vi "Wait for Response Message.vi"(8 "error in (no error)":errorcluster, 9 "timeout in ms":i32, 11 "Process in":refnum<class "Process.lvclass">) -> (0 "error out":errorcluster, 1 "Message Data":variant, 2 "Message":string, 3 "Process out":refnum<class "Process.lvclass">, 4 "timed out?":bool)   [LabVIEW 2020, in "Process.lvclass"]
uses:
  Process.lvclass
  Process.lvclass/Process.ctl
  <vilib>/Utility/error.llb/Error Cluster From Error Code.vi
  <vilib>/ErrorRing/Error Ring.xnode
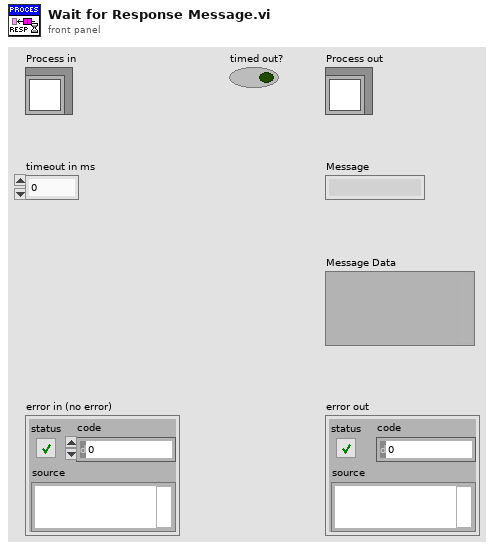
[diagram p1: front panel]
types:
  T1 = typedef "Process.lvclass/Lifecycle State.ctl" = enum16{"Uninitialized", "Initialized", "Started", "Running", "Stopped", "Finished"}
  T2 = typedef "Process.lvclass/Request Message Cluster.ctl" = cluster{"Message":string, "Message Data":variant}
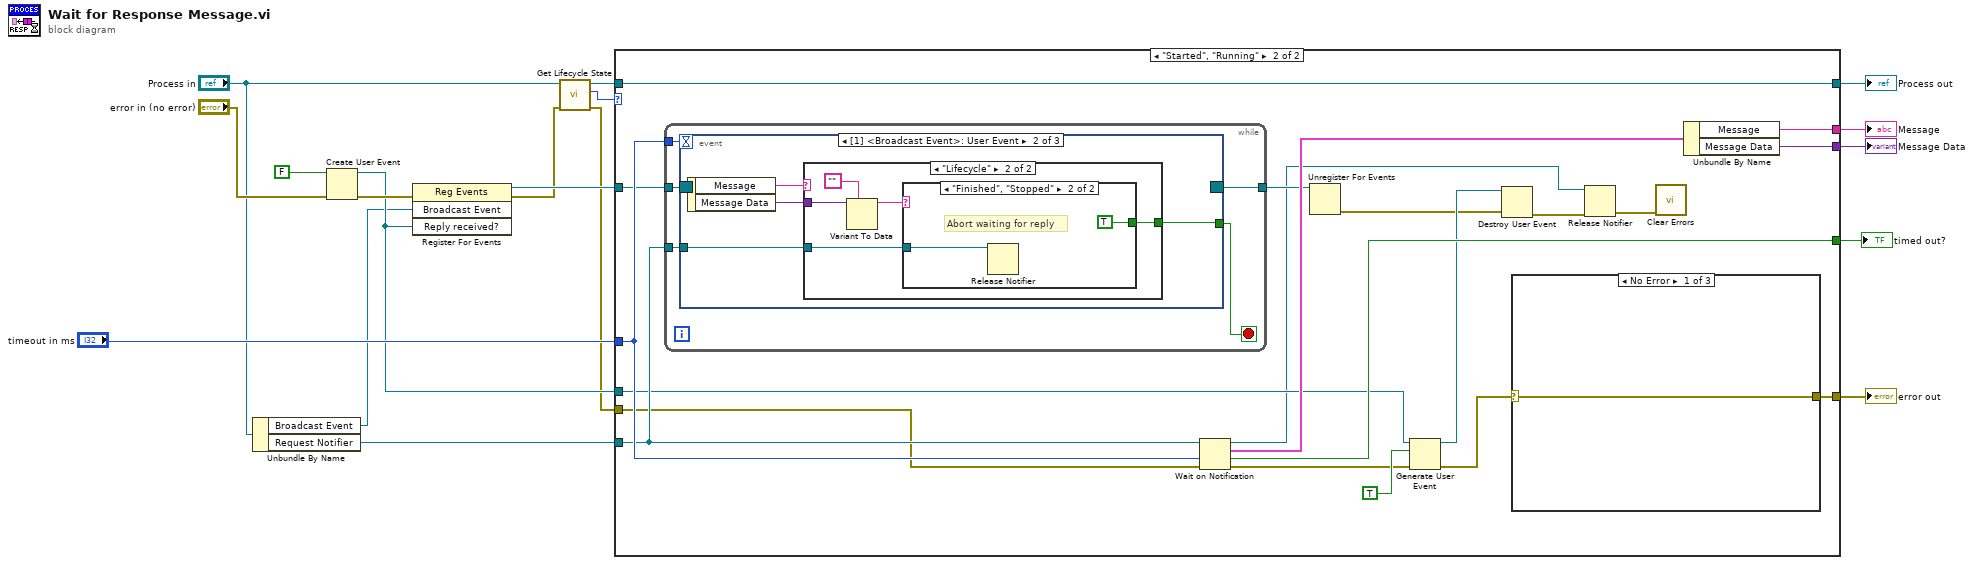
[diagram p0: block diagram]
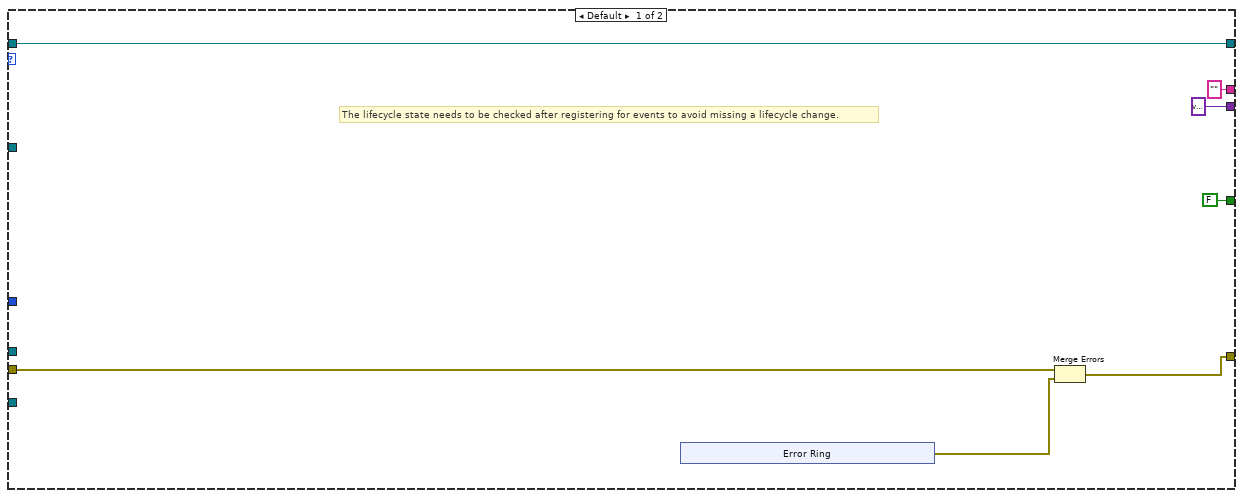
[diagram p2: hidden frame]
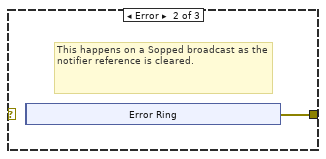
[diagram p3: hidden frame]
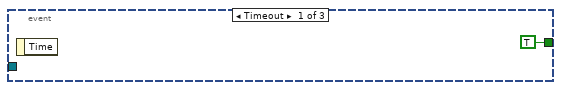
[diagram p5: hidden frame]
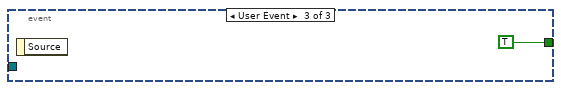
[diagram p8: hidden frame]
diagram:
  n1 = Unbundle By Name("Process in") -> ("Broadcast Event"=w6:refnum<user-event>, "Request Notifier"=w9:refnum<notifier>)
  n2 = Create User Event(user event datatype=FALSE ("Reply received?"), error in="error in (no error)") -> (user event=w7:refnum<user-event>, error out=w17:errorcluster)
  n3 = register-events(error in=w17, w6, w7) -> (reference out=w14:refnum<event-registration>, error out=w5:errorcluster)  [unwired: 1 in]
  n4 = call "Get Lifecycle State.vi"("error in (no error)"=w5, "Process In"="Process in") -> ("error out"=w4:errorcluster, "Lifecycle State"=w1:T1, "Process Out"=w2:refnum<class "Process.lvclass">)  [unwired: 6 in, 1 out]
  n5 = case shown="\"Started\", \"Running\"" w1 {
    tunnel: "timeout in ms" -> [_ w49]
    tunnel: w14 -> [_ w48]
    tunnel: [variant ("Message Data") w47] -> w13
    tunnel: ["" ("Message") w46] -> w12
    tunnel: [FALSE ("timed out?") w44] -> w11
    tunnel: w9 -> [_ w43]
    tunnel: [w23 w41] -> w8
    tunnel: w7 -> [_ w39]
    tunnel: w4 -> [w24 w31]
    tunnel: [w25 w30] -> w3
    tunnel: w2 -> [w25 w30]
    frame Default {
      # "The lifecycle state needs to be checked after registering for events to avoid missing a lifecycle change."
      n6 = xnode "Error Ring"() -> ("error out"=w22:errorcluster)
      n7 = Merge Errors(w24, w22) -> (w23:errorcluster)
    }
    frame "Started", "Running" {
      n8 = while {
        tunnel: w48 -> [w65]
        tunnel: w49 -> [w64]
        tunnel: w43 -> [w62]
        tunnel: [w61] -> w42
        stop <- w63 stop-if-true
        n9 = event shown="[1] <Broadcast Event>: User Event" {
          selector: w65 -> [_ _ _]
          dyn-events: [_ _ _] -> w61
          timeout: w64 -> [_ _ _]
          tunnel: [TRUE w67 TRUE] -> w63
          tunnel: w62 -> [_ w68 _]
          event Timeout {
            n10 = event-data() -> ()  [unwired: 1 in, 1 out]
          }
          event User Event {
            n11 = event-data() -> ("Message"=w70:string, "Message Data"=w69:variant)  [unwired: 1 in]
            n12 = case shown="\"Lifecycle\"" w70 {
              tunnel: w69 -> [_ w75]
              tunnel: w68 -> [_ w72]
              tunnel: [_ w71] -> w67
              frame Default {
              }
              frame "Lifecycle" {
                n13 = Variant To Data(type="", Variant=w75) -> (data=w73:string)  [unwired: 1 in, 1 out]
                n14 = case shown="\"Finished\", \"Stopped\"" w73 {
                  tunnel: w72 -> [_ w77]
                  tunnel: [_ TRUE] -> w71
                  frame Default {
                  }
                  frame "Finished", "Stopped" {
                    # "Abort waiting for reply"
                    n15 = Release Notifier(notifier=w77) -> ()  [unwired: 2 in, 3 out]
                  }
                }
              }
            }
          }
          event User Event {
            n16 = event-data() -> ()  [unwired: 1 in, 1 out]
          }
        }
      }
      n17 = Wait on Notification(notifier=w43, timeout in ms (-1)=w49, error in (no error)=w31) -> (notifier out=w33:refnum<notifier>, notification=w45:T2, timed out?=w44:bool, error out=w35:errorcluster)  [unwired: 1 in]
      n18 = Unregister For Events(event registration refnum=w42) -> (error out=w37:errorcluster)  [unwired: 1 in]
      n19 = Generate User Event(user event=w39, event data cluster=TRUE ("event data"), error in=w35) -> (user event out=w38:refnum<user-event>, error out=w40:errorcluster)  [unwired: 1 in]
      n20 = Destroy User Event(user event=w38, error in=w37) -> (error out=w34:errorcluster)
      n21 = case shown="No Error" w40 {
        selector: w40 -> [w50 _ w60]
        tunnel: [w50 w51 w60] -> w41
        frame No Error {
        }
        frame Error {
          # "This happens on a Sopped broadcast as the notifier reference is cleared."
          n22 = xnode "Error Ring"() -> ()  [unwired: 1 out]
          n23 = xnode "Error Ring"() -> ("error out"=w51:errorcluster)
        }
        frame Default {
        }
      }
      n24 = Release Notifier(notifier=w33, error in (no error)=w34) -> (error out=w32:errorcluster)  [unwired: 1 in, 2 out]
      n25 = call <vilib>:"Clear Errors.vi"("error in (no error)"=w32) -> ()  [unwired: 5 in, 2 out]
      n26 = Unbundle By Name(w45) -> ("Message"=w46:string, "Message Data"=w47:variant)
    }
  }
  "Process out" <- w3
  "error out" <- w8
  "Message Data" <- w13
  "Message" <- w12
  "timed out?" <- w11
